vi "Request_Update Items.vi"(8 "error in":errorcluster, 11 "Changed Items":T1) -> (0 "error out":errorcluster)   [LabVIEW 2013, in "LVTM.lvlib"]
doc: "This allows for initiating a pause from within any VI on some condition. Just drop this VI in a case structure after your custom probe condition evaluation. It will only work if the task manager is open. If the pause request is generated from a clone of a reentrant VI, it will pause all clones of that VI.\n\n<b>Note that the User Event terminals are used only internally, and should NOT be wired for normal use.</b>"
uses:
  LVTM.lvlib
  Controls_LVTM/UserEventUpdateTreeItems.ctl
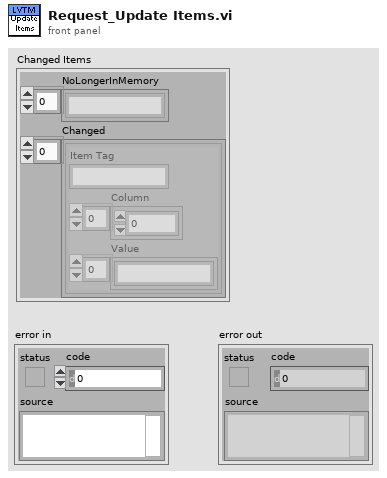
[diagram p1: front panel]
types:
  T1 = typedef "LVTM.lvlib/UserEventUpdateTreeItems.ctl" = cluster{"NoLongerInMemory":string[], "Changed":cluster{"Item Tag":string, "Column":i32[], "Value":string[]}[]}
  T2 = typedef "LVTM.lvlib/RequestEvents.ctl" = cluster{"Pause":refnum<user-event>, "Handle Error":refnum<user-event>, "Update Items":refnum<user-event>}
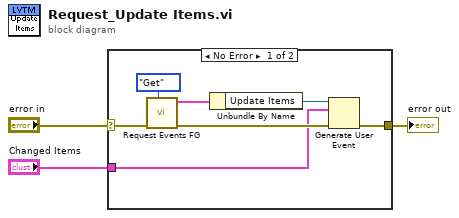
[diagram p0: block diagram]
diagram:
  n1 = case shown="No Error" "error in" {
    selector: "error in" -> [w5 w11]
    tunnel: [w7 w11] -> w3
    tunnel: "Changed Items" -> [w4 _]
    frame No Error {
      n2 = call "Request Events FG.vi"("Action (Get)"=enum16{"Initialize", "Get", "Destroy"}."Get" ("Action"), "error in"=w5) -> ("error out"=w6:errorcluster, "Request Events"=w9:T2)  [unwired: 8 in]
      n3 = Unbundle By Name(w9) -> ("Update Items"=w8:refnum<user-event>)
      n4 = Generate User Event(user event=w8, event data cluster=w4, error in=w6) -> (error out=w7:errorcluster)  [unwired: 1 in, 1 out]
    }
    frame Error {
    }
  }
  "error out" <- w3
